vi "Begin.vi"(11 "Image Size":T1) -> (0 "error out":errorcluster)   [LabVIEW 2011]
doc: "Called before other user functions, this VI is expected to open initial I/O refnums, load in file data, and do all program initialization. Notice that the <B>error out</B> terminal is simply used for data flow. Wiring it to other structures or subVIs ensures that this VI runs first."
uses:
  <vilib>/Rock Robotics/WPI/Camera/WPI_CameraImageSize.ctl
  <vilib>/Rock Robotics/WPI/Joystick/WPI_JoystickDeviceEnum.ctl
  <vilib>/Rock Robotics/WPI/Camera/WPI_CameraWhite Balance Values.ctl
  <vilib>/Rock Robotics/WPI/Camera/WPI_CameraExposure Values.ctl
  <vilib>/Rock Robotics/WPI/Camera/WPI_CameraFrameRate.ctl
  <vilib>/Rock Robotics/SystemInterfaces/DIO/FPGA_DIOPWMChannel.ctl
  <vilib>/Rock Robotics/SystemInterfaces/Typedef/FPGA_TypedefAnalogModule.ctl
  <vilib>/Rock Robotics/SystemInterfaces/AI/FPGA_AIChannel.ctl
  <vilib>/Rock Robotics/SystemInterfaces/Typedef/FPGA_TypedefDigitalModule.ctl
  <vilib>/Rock Robotics/SystemInterfaces/DIO/FPGA_DIORelayChannel.ctl
  <vilib>/Rock Robotics/WPI/Relay/WPI_RelayDirection.ctl
  <vilib>/Rock Robotics/WPI/MotorControl/WPI_MotorControlOpen Victor.vi
  <vilib>/Rock Robotics/WPI/RobotDrive/WPI_RobotDriveOpen2MotorWithVictor.vi
  <vilib>/Rock Robotics/SystemInterfaces/Typedef/FPGA_TypedefAnalogModuleForGyro.ctl
  <vilib>/Rock Robotics/SystemInterfaces/AI/FPGA_AIGyroChannel.ctl
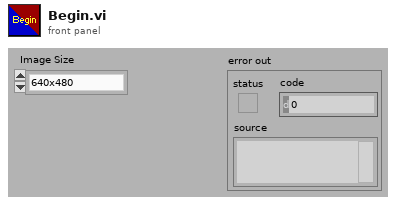
[diagram p1: front panel]
types:
  T1 = typedef "WPI_CameraImageSize.ctl" = enum16{"640x480", "320x240", "160x120"}
  T2 = typedef "WPI_RelayDirection.ctl" = enum16{"Both directions", "Forward only", "Reverse only"}
  T3 = typedef "FPGA_DIORelayChannel.ctl" = enum8{"Relay 1", "Relay 2", "Relay 3", "Relay 4", "Relay 5", "Relay 6", "Relay 7", "Relay 8", "Invalid"}
  T4 = typedef "FPGA_TypedefDigitalModule.ctl" = enum16{"Digital Module 1", "Digital Module 2"}
  T5 = typedef "FPGA_AIChannel.ctl" = enum8{"AI 1", "AI 2", "AI 3", "AI 4", "AI 5", "AI 6", "AI 7", "AI 8", "Invalid"}
  T6 = typedef "FPGA_TypedefAnalogModule.ctl" = enum16{"Analog Module 1", "Analog Module 2"}
  T7 = typedef "WPI_JoystickDeviceEnum.ctl" = enum16{"USB 1", "USB 2", "USB 3", "USB 4", "Kinect 1", "Kinect 2"}
  T8 = typedef "FPGA_DIOPWMChannel.ctl" = enum8{"PWM 1", "PWM 2", "PWM 3", "PWM 4", "PWM 5", "PWM 6", "PWM 7", "PWM 8", "PWM 9", "PWM 10", "Invalid"}
  T9 = typedef "WPI_CameraFrameRate.ctl" = u32
  T10 = typedef "WPI_CameraExposure Values.ctl" = enum16{"Auto", "Flicker-free 50 Hz", "Flicker-free 60 Hz", "Hold current"}
  T11 = typedef "WPI_CameraWhite Balance Values.ctl" = enum16{"Auto", "Fixed indoor", "Fixed outdoor 1", "Fixed outdoor 2", "Fixed fluorescent 1", "Fixed fluorescent 2", "Hold current"}
  T12 = typedef "WPI_ServoDeviceRef.ctl" = cluster{"DeviceStatus":errorcluster, "Digital Module":T4, "PWM Channel":T8, "DeadBand":T13}
  T13 = typedef "WPI_PWMDeadband.ctl" = cluster{"Name":string, "maxPositivePwm":i32, "minPositivePwm":i32, "centerPwm":i32, "maxNegativePwm":i32, "minNegativePwm":i32, "angularRange":u16}
  T14 = typedef "WPI_MotorControlDeviceRef.ctl" = cluster{"DeviceStatus":errorcluster, "Type":enum16{"PWM", "CAN"}, "PWM":cluster{"Digital Module":T4, "PWM Channel":T8, "DeadBand":T13}, "CAN":cluster{"Device Number":u8, "Control Mode":T15, "Semaphore":T16, "Max Vout":dbl}, "Invert":bool, "TransformRef":T17, "InvTransformRef":T17}
  T15 = typedef "WPI_CANJaguar_ControlMode.ctl" = enum8{"Percent VBus", "Current", "Speed", "Position", "Voltage"}
  T16 = typedef "Semaphore RefNum" = refnum<k1>
  T17 = typedef "WPI_PWMTransform_ConPane.ctl" = refnum<vi>
  T18 = typedef "WPI_RobotDriveDevRef.ctl" = cluster{"DevStatus":errorcluster, "Motors[]":T14[], "Square Inputs":bool, "Max Output":dbl, "Isochronous":bool}
  T19 = typedef "WPI_JoystickDevRef.ctl" = cluster{"Device":T7}
  T20 = typedef "WPI_RelayDevRef.ctl" = cluster{"DevStatus":errorcluster, "Relay Channel":T3, "Digital Module":T4, "Relay Direction":T2}
  T21 = typedef "WPI_CameraDevRef.ctl" = cluster{"Camera Address":string, "CameraStatus":errorcluster, "Acquire Image Notifier":refnum<notifier>}
  T22 = typedef "FPGA_AIGyroChannel.ctl" = enum8{"AI 1", "AI 2", "Invalid"}
  T23 = typedef "FPGA_TypedefAnalogModuleForGyro.ctl" = enum16{"Analog Module 1"}
  T24 = typedef "WPI_AccelerometerDevRef.ctl" = cluster{"DevStatus":errorcluster, "Analog Module":T6, "Analog Channel":T5, "Scaling":T25}
  T25 = typedef "WPI_AccelerometerScaling.ctl" = cluster{"Gain (VoltsPerG)":dbl, "Center Voltage":dbl}
  T26 = typedef "WPI_GyroDevRef.ctl" = cluster{"DevStatus":errorcluster, "Analog Module":T6, "Analog Channel":T5, "Offset":dbl, "Gain (VoltsPerDegree/Second)":dbl}
  T27 = typedef "WPI_AnalogChannelDevRef.ctl" = cluster{"DevStatus":errorcluster, "Analog Module":T6, "Analog Channel":T5}
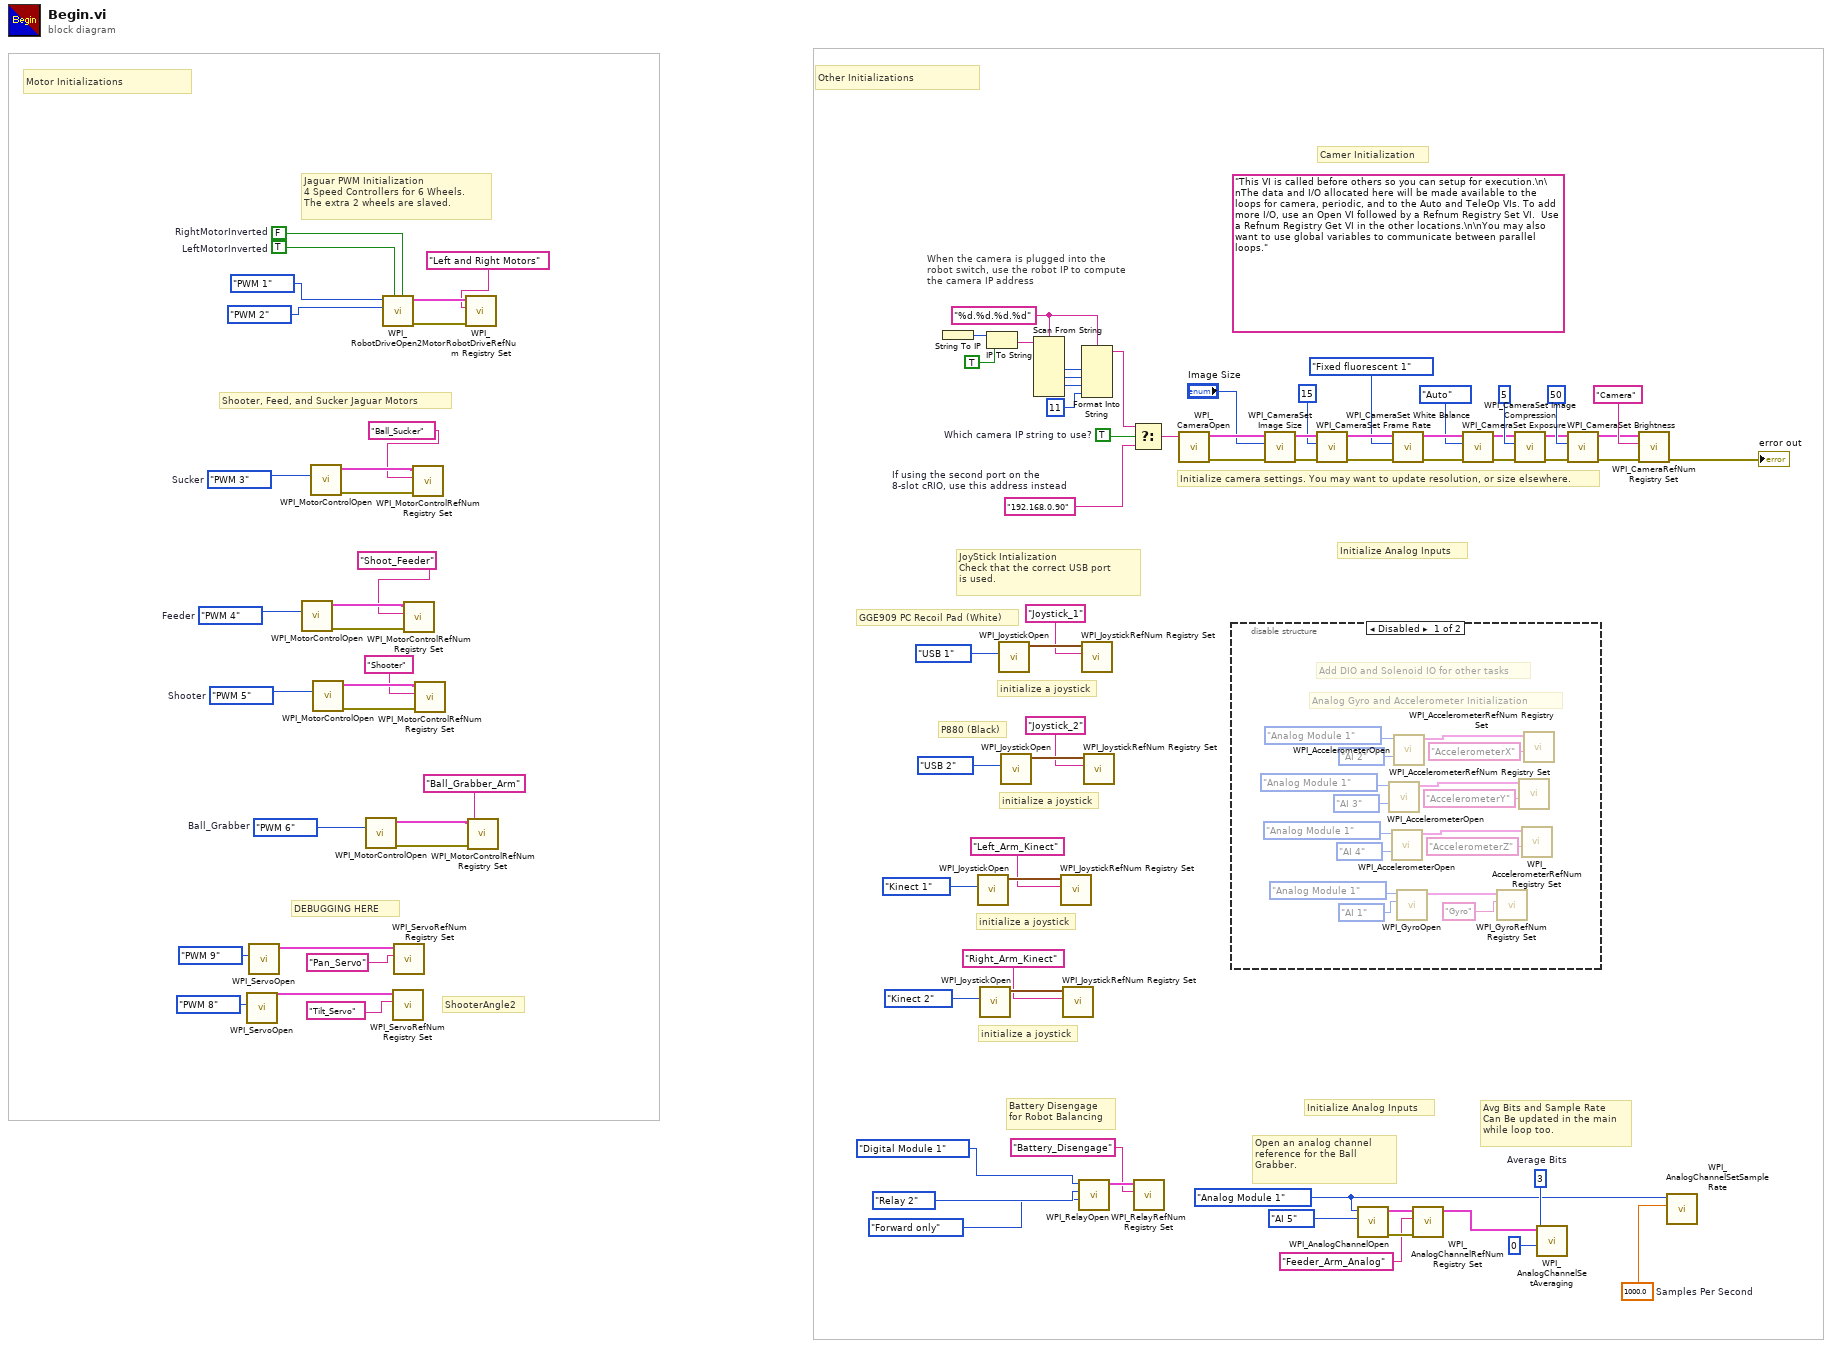
[diagram p0: block diagram]
diagram:
  w14 = 1000.0  # Samples Per Second
  w13 = u8 3  # Average Bits
  w12 = FPGA_TypedefAnalogModule."Analog Module 1" ("Analog Module (Slot 1)")
  w24 = FPGA_DIOPWMChannel."PWM 6"  # Ball_Grabber
  w32 = TRUE  # LeftMotorInverted
  w33 = FALSE  # RightMotorInverted
  w41 = FPGA_DIOPWMChannel."PWM 5"  # Shooter
  w45 = FPGA_DIOPWMChannel."PWM 4"  # Feeder
  w49 = FPGA_DIOPWMChannel."PWM 3"  # Sucker
  w54 = TRUE  # Which camera IP string to use?
  w58 = "%d.%d.%d.%d" ("format string")
  (unwired) "This VI is called before others so you can setup for execution.\n\nThe data and I/O allocated here will be made available to the loops for camera, periodic, and to the Auto and TeleOp VIs. To add more I/O, use an Open VI followed by a Refnum Registry Set VI.  Use a Refnum Registry Get VI in the other locations.\n\nYou may also want to use global variables to communicate between parallel loops."
  w55 = "192.168.0.90"  # If using the second port on the 8-slot cRIO, use this address instead
  # "Battery Disengage \nfor Robot Balancing"
  # "Avg Bits and Sample Rate\nCan Be updated in the main\nwhile loop too."
  # "Open an analog channel reference for the Ball Grabber."
  # "Initialize Analog Inputs"
  # "P880 (Black)"
  # "GGE909 PC Recoil Pad (White)"
  # "initialize a joystick"
  # "initialize a joystick"
  # "Initialize Analog Inputs"
  # "DEBUGGING HERE"
  # "Other Initializations"
  # "Motor Initializations"
  # "Shooter, Feed, and Sucker Jaguar Motors"
  # "Jaguar PWM Initialization\n4 Speed Controllers for 6 Wheels.\nThe extra 2 wheels are slaved."
  # "JoyStick Intialization\nCheck that the correct USB port\nis used."
  # "Camer Initialization"
  # "ShooterAngle2"
  # "initialize a joystick"
  # "When the camera is plugged into the\nrobot switch, use the robot IP to compute\nthe camera IP address"
  # "initialize a joystick"
  # "Initialize camera settings. You may want to update resolution, or size elsewhere."
  n1 = call <vilib>:"WPI_ServoOpen.vi"("PWM Channel"=FPGA_DIOPWMChannel."PWM 8") -> ("ServoDeviceRef"=w29:T12)  [unwired: 3 in, 7 out]
  n2 = call <vilib>:"WPI_ServoOpen.vi"("PWM Channel"=FPGA_DIOPWMChannel."PWM 9") -> ("ServoDeviceRef"=w31:T12)  [unwired: 3 in, 7 out]
  n3 = call-poly <vilib>:"WPI_MotorControlOpen.vi"("PWM Channel"=w45) -> ("error out"=w46:errorcluster, "MotorControlDeviceRef"=w44:T14)  [unwired: 9 in]
  n4 = call-poly <vilib>:"WPI_MotorControlOpen.vi"("PWM Channel"=w49) -> ("error out"=w50:errorcluster, "MotorControlDeviceRef"=w48:T14)  [unwired: 9 in]
  n5 = call-poly <vilib>:"WPI_MotorControlOpen.vi"("PWM Channel"=w41) -> ("error out"=w42:errorcluster, "MotorControlDeviceRef"=w40:T14)  [unwired: 9 in]
  n6 = call-poly <vilib>:"WPI_MotorControlOpen.vi"("PWM Channel"=w24) -> ("error out"=w26:errorcluster, "MotorControlDeviceRef"=w25:T14)  [unwired: 9 in]
  n7 = call-poly <vilib>:"WPI_RobotDriveOpen2Motor.vi"("Right Motor Inverted"=w33, "Left Motor Inverted"=w32, "Right Motor"=FPGA_DIOPWMChannel."PWM 2" ("RearRightMotor"), "Left Motor"=FPGA_DIOPWMChannel."PWM 1" ("RearLeftMotor")) -> ("error out"=w38:errorcluster, "RobotDriveDevRef"=w37:T18)  [unwired: 6 in]
  n8 = call <vilib>:"WPI_ServoRefNum Registry Set.vi"("refnum name"="Tilt_Servo", "ServoDeviceRef"=w29) -> ()  [unwired: 1 in, 9 out]
  n9 = call <vilib>:"WPI_ServoRefNum Registry Set.vi"("refnum name"="Pan_Servo", "ServoDeviceRef"=w31) -> ()  [unwired: 1 in, 9 out]
  n10 = call <vilib>:"WPI_MotorControlRefNum Registry Set.vi"("error in (no error)"=w46, "refnum name"="Shoot_Feeder", "MotorControlDevRef"=w44) -> ()  [unwired: 7 in, 2 out]
  n11 = call <vilib>:"WPI_MotorControlRefNum Registry Set.vi"("error in (no error)"=w50, "refnum name"="Ball_Sucker", "MotorControlDevRef"=w48) -> ()  [unwired: 7 in, 2 out]
  n12 = call <vilib>:"WPI_MotorControlRefNum Registry Set.vi"("error in (no error)"=w42, "refnum name"="Shooter", "MotorControlDevRef"=w40) -> ()  [unwired: 7 in, 2 out]
  n13 = call <vilib>:"WPI_RobotDriveRefNum Registry Set.vi"("error in (no error)"=w38, "refnum name"="Left and Right Motors", "RobotDriveDevRef"=w37) -> ()  [unwired: 9 out]
  n14 = call <vilib>:"WPI_MotorControlRefNum Registry Set.vi"("error in (no error)"=w26, "refnum name"="Ball_Grabber_Arm", "MotorControlDevRef"=w25) -> ()  [unwired: 7 in, 2 out]
  n15 = String To IP() -> (0:w65:u32)  [unwired: 1 in]
  n16 = call <vilib>:"WPI_JoystickOpen.vi"("JoystickDevice"=WPI_JoystickDeviceEnum."Kinect 1") -> ("JoystickDevRef"=w22:T19)  [unwired: 10 out]
  n17 = call <vilib>:"WPI_JoystickOpen.vi"("JoystickDevice"=WPI_JoystickDeviceEnum."Kinect 2") -> ("JoystickDevRef"=w19:T19)  [unwired: 10 out]
  n18 = IP To String(1:TRUE ("dot notation? (F)"), 2:w65) -> (0:w63:string)
  n19 = call <vilib>:"WPI_JoystickOpen.vi"("JoystickDevice"=WPI_JoystickDeviceEnum."USB 1") -> ("JoystickDevRef"=w88:T19)  [unwired: 10 out]
  n20 = call <vilib>:"WPI_JoystickOpen.vi"("JoystickDevice"=WPI_JoystickDeviceEnum."USB 2") -> ("JoystickDevRef"=w53:T19)  [unwired: 10 out]
  n21 = Scan From String(format string=w58, input string=w63) -> (output 1=w62:i32, output 2=w61:i32, output 3=w60:i32)  [unwired: 7 in, 3 out]
  n22 = call <vilib>:"WPI_JoystickRefNum Registry Set.vi"("refnum name"="Left_Arm_Kinect", "JoystickDevRef"=w22) -> ()  [unwired: 1 in, 9 out]
  n23 = call <vilib>:"WPI_JoystickRefNum Registry Set.vi"("refnum name"="Right_Arm_Kinect", "JoystickDevRef"=w19) -> ()  [unwired: 1 in, 9 out]
  n24 = call <vilib>:"WPI_RelayOpen.vi"("Relay Direction"=WPI_RelayDirection."Forward only" ("RelayDirection"), "Relay Channel"=FPGA_DIORelayChannel."Relay 2" ("RelayChannel"), "Digital Module (Module 1)"=FPGA_TypedefDigitalModule."Digital Module 1" ("DIO Module")) -> ("RelayDevRef"=w2:T20)  [unwired: 1 in, 7 out]
  n25 = Format Into String(format string=w58, w62, w61, w60, 11 ("Compression")) -> (resulting string=w56:string)  [unwired: 2 in, 1 out]
  n26 = call <vilib>:"WPI_JoystickRefNum Registry Set.vi"("refnum name"="Joystick_1", "JoystickDevRef"=w88) -> ()  [unwired: 1 in, 9 out]
  n27 = call <vilib>:"WPI_JoystickRefNum Registry Set.vi"("refnum name"="Joystick_2", "JoystickDevRef"=w53) -> ()  [unwired: 1 in, 9 out]
  n28 = Select(t=w56, s=w54, f=w55) -> (s? t:f=w57:string)
  n29 = call <vilib>:"WPI_RelayRefNum Registry Set.vi"("refnum name"="Battery_Disengage", "RelayDevRef"=w2) -> ()  [unwired: 8 in, 2 out]
  n30 = call <vilib>:"WPI_CameraOpen.vi"("Camera Address"=w57) -> ("error out"=w78:errorcluster, "CameraDevRef"=w79:T21)  [unwired: 1 in, 8 out]
  n31 = disable-structure shown="Disabled" {
    frame Disabled {
      # "Add DIO and Solenoid IO for other tasks"
      # "Analog Gyro and Accelerometer Initialization"
      n32 = call <vilib>:"WPI_AccelerometerOpen.vi"("Analog Channel"=FPGA_AIChannel."AI 3", "Analog Module (Module 1)"=FPGA_TypedefAnalogModule."Analog Module 1" ("Analog Module (Slot 1)")) -> ("AccelerometerDevRef"=w96:T24)  [unwired: 2 in, 7 out]
      n33 = call <vilib>:"WPI_AccelerometerOpen.vi"("Analog Channel"=FPGA_AIChannel."AI 4", "Analog Module (Module 1)"=FPGA_TypedefAnalogModule."Analog Module 1" ("Analog Module (Slot 1)")) -> ("AccelerometerDevRef"=w93:T24)  [unwired: 2 in, 7 out]
      n34 = call <vilib>:"WPI_AccelerometerOpen.vi"("Analog Channel"=FPGA_AIChannel."AI 2", "Analog Module (Module 1)"=FPGA_TypedefAnalogModule."Analog Module 1" ("Analog Module (Slot 1)")) -> ("AccelerometerDevRef"=w101:T24)  [unwired: 2 in, 7 out]
      n35 = call <vilib>:"WPI_GyroOpen.vi"("Analog Channel"=FPGA_AIGyroChannel."AI 1", "Analog Module (Module 1)"=FPGA_TypedefAnalogModuleForGyro."Analog Module 1" ("Analog Module (Slot 1)")) -> ("GyroDevRef"=w103:T26)  [unwired: 4 in, 5 out]
      n36 = call <vilib>:"WPI_GyroRefNum Registry Set.vi"("refnum name"="Gyro", "GyroDevRef"=w103) -> ()  [unwired: 1 in, 9 out]
      n37 = call <vilib>:"WPI_AccelerometerRefNum Registry Set.vi"("refnum name"="AccelerometerY", "AccelerometerDevRef"=w96) -> ()  [unwired: 1 in, 9 out]
      n38 = call <vilib>:"WPI_AccelerometerRefNum Registry Set.vi"("refnum name"="AccelerometerZ", "AccelerometerDevRef"=w93) -> ()  [unwired: 1 in, 9 out]
      n39 = call <vilib>:"WPI_AccelerometerRefNum Registry Set.vi"("refnum name"="AccelerometerX", "AccelerometerDevRef"=w101) -> ()  [unwired: 1 in, 9 out]
    }
    frame Enabled {
    }
  }
  n40 = call <vilib>:"WPI_CameraSet Image Size.vi"("error in (no error)"=w78, "Image Size"="Image Size", "CameraDevRef"=w79) -> ("error out"=w77:errorcluster, "CameraDevRef Out"=w80:T21)  [unwired: 7 out]
  n41 = call <vilib>:"WPI_CameraSet Frame Rate.vi"("error in (no error)"=w77, "Frame Rate (fps)"=T9 15, "CameraDevRef"=w80) -> ("error out"=w76:errorcluster, "CameraDevRef Out"=w82:T21)  [unwired: 7 out]
  n42 = call <vilib>:"WPI_AnalogChannelOpen.vi"("Analog Channel"=FPGA_AIChannel."AI 5", "Analog Module (Module 1)"=w12) -> ("error out"=w11:errorcluster, "AIDeviceRef"=w10:T27)  [unwired: 1 in, 7 out]
  n43 = call <vilib>:"WPI_CameraSet White Balance.vi"("error in (no error)"=w76, "White Balance"=WPI_CameraWhite_Balance_Values."Fixed fluorescent 1", "CameraDevRef"=w82) -> ("error out"=w75:errorcluster, "CameraDevRef Out"=w81:T21)  [unwired: 7 out]
  n44 = call <vilib>:"WPI_AnalogChannelRefNum Registry Set.vi"("error in (no error)"=w11, "refnum name"="Feeder_Arm_Analog", "AIDeviceRef"=w10) -> ("AIDeviceRef"=w9:T27)  [unwired: 7 in, 1 out]
  n45 = call <vilib>:"WPI_CameraSet Exposure.vi"("error in (no error)"=w75, "Exposure"=WPI_CameraExposure_Values."Auto", "CameraDevRef"=w81) -> ("error out"=w74:errorcluster, "CameraDevRef Out"=w84:T21)  [unwired: 7 out]
  n46 = call <vilib>:"WPI_CameraSet Image Compression.vi"("error in (no error)"=w74, "Compression"=5, "CameraDevRef"=w84) -> ("error out"=w73:errorcluster, "CameraDevRef Out"=w83:T21)  [unwired: 7 out]
  n47 = call <vilib>:"WPI_AnalogChannelSetAveraging.vi"("OversampleBits"=u8 0, "AverageBits"=w13, "AIDeviceRef"=w9) -> ()  [unwired: 1 in, 8 out]
  n48 = call <vilib>:"WPI_CameraSet Brightness.vi"("error in (no error)"=w73, "Brightness"=50, "CameraDevRef"=w83) -> ("error out"=w71:errorcluster, "CameraDevRef Out"=w72:T21)  [unwired: 7 out]
  n49 = call <vilib>:"WPI_CameraRefNum Registry Set.vi"("error in (no error)"=w71, "refnum name"="Camera", "CameraDevRef"=w72) -> ("error out"=→"error out":errorcluster)  [unwired: 8 out]
  n50 = call <vilib>:"WPI_AnalogChannelSetSampleRate.vi"("Samples Per Second"=w14, "Analog Module (Module 1)"=w12) -> ()  [unwired: 2 in, 8 out]
